vi "Dyn - State To Execute.vi"(0 "LVx Command in":refnum<class "LVx.lvclass">, 11 "error in (no error)":errorcluster) -> (4 "LVx Command out":refnum<class "LVx.lvclass">, 8 "State To Execute":string, 15 "error out":errorcluster)   [LabVIEW 2011, in "LVx.lvlib" / "LVx.lvclass"]
uses:
  LVx.lvclass
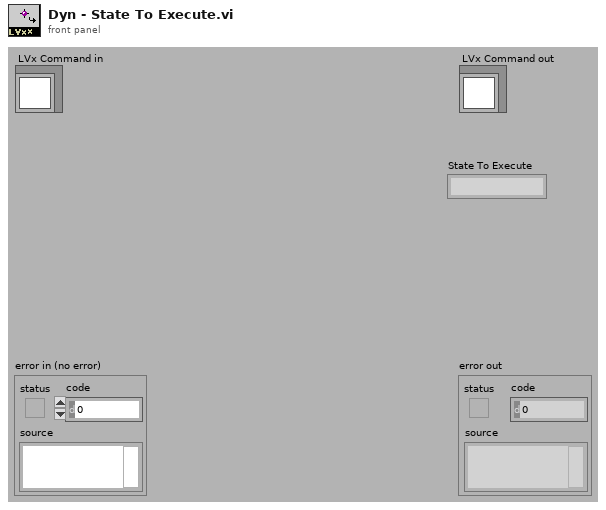
[diagram p1: front panel]
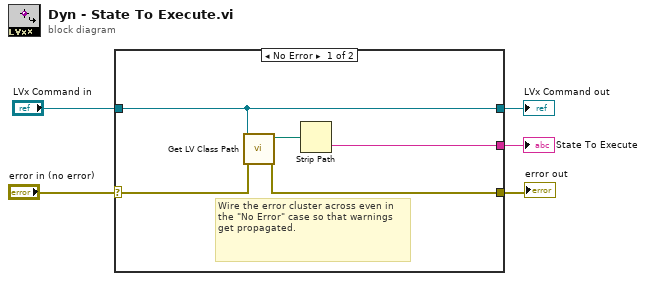
[diagram p0: block diagram]
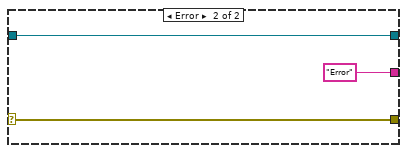
[diagram p2: hidden frame]
diagram:
  n1 = case shown="No Error" "error in (no error)" {
    selector: "error in (no error)" -> [w8 w13]
    tunnel: [w7 w13] -> w4
    tunnel: [w10 w12] -> w2
    tunnel: "LVx Command in" -> [w10 w12]
    tunnel: [w9 "Error" ("State To Execute")] -> w1
    frame No Error {
      # "Wire the error cluster across even in the \"No Error\" case so that warnings get propagated."
      n2 = call <vilib>:"Get LV Class Path.vi"("error in (no error)"=w8, "object"=w10) -> ("error out"=w7:errorcluster, "class path"=w6:path)  [unwired: 8 in]
      n3 = Strip Path(path=w6) -> (name=w9:string)  [unwired: 1 out]
    }
    frame Error {
    }
  }
  "error out" <- w4
  "LVx Command out" <- w2
  "State To Execute" <- w1
